vi "Decode Tags.vi"(11 "Tags in":u8) -> (1 "Echo out":bool, 2 "Extended ID":bool, 3 "ISO FD Type":T1=enum."CAN 2.0")   [LabVIEW 2021, in "CAN_Logic.lvclass"]
uses:
  CAN_Logic.lvclass
  typedef/ISO FD Frame Type.ctl
  CAN_Logic.lvclass/CAN_Logic.ctl
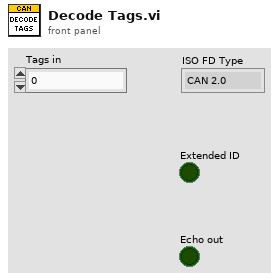
[diagram p1: front panel]
types:
  T1 = typedef "CAN_Logic.lvclass/ISO FD Frame Type.ctl" = enum16{"Not Specified", "CAN 2.0", "FD", "FD+BRS"}
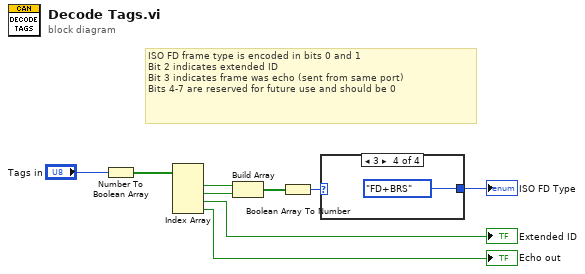
[diagram p0: block diagram]
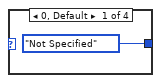
[diagram p2: hidden frame]
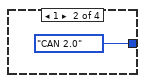
[diagram p3: hidden frame]
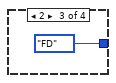
[diagram p4: hidden frame]
diagram:
  # "ISO FD frame type is encoded in bits 0 and 1\nBit 2 indicates extended ID\nBit 3 indicates frame was echo (sent from same port)\nBits 4-7 are reserved for future use and should be 0"
  n1 = Number To Boolean Array(number="Tags in") -> (Boolean array=w9:bool[])
  n2 = Index Array(array=w9) -> (element #1=w6:bool, element #2=w5:bool, element #3=→"Extended ID":bool, element #4=→"Echo out":bool)  [unwired: 4 in]
  n3 = Build Array(w6, w5) -> (w4:bool[])
  n4 = Boolean Array To Number(Boolean array=w4) -> (number=w3:u8)
  n5 = case shown="3" w3 {
    tunnel: [ISO_FD_Frame_Type."Not Specified" ("ISO FD Type 2") ISO_FD_Frame_Type."CAN 2.0" ("ISO FD Type 2") ISO_FD_Frame_Type."FD" ("ISO FD Type 2") ISO_FD_Frame_Type."FD+BRS" ("ISO FD Type 2")] -> w2
    frame 0, Default {
    }
    frame 1 {
    }
    frame 2 {
    }
    frame 3 {
    }
  }
  "ISO FD Type" <- w2
